vi "Configure Multi Eval Meas Modulation EVM Window Length.vi"(7 "SCS 120kHz":i32[](array[numeric]), 8 "error in (no error)":errorcluster, 9 "SCS 60kHz":i32[](array[numeric]), 10 "Instance (1)":T1=1, 11 "VISA resource name":refnum<visa-resource-name>) -> (0 "error out":errorcluster, 3 "VISA resource name out":refnum<visa-resource-name>)   [LabVIEW 2020, in "Rohde&Schwarz CMXP NR FR2 Measurement.lvlib"]
doc: "Specifies the EVM window length in samples for all channel bandwidths, depending on the SC spacing.\n\nAttribute:\nRSCMXPNRFR2M_ATTR_MULTI_EVAL_MEASUREMENT_MODULATION_EVM_WINDOW_LENGTH\n\nRemote-control command:\nCONFigure:NRMMw:MEAS<i>:MEValuation:MODulation:EWLength"
uses:
  <instrlib>/Rohde&Schwarz CMXP NR FR2 Measurement/Rohde&Schwarz CMXP NR FR2 Measurement.lvlib
  <instrlib>/Rohde&Schwarz CMXP NR FR2 Measurement/Private/_Instance.ctl
  <instrlib>/Rohde&Schwarz CMXP NR FR2 Measurement/Private/rsidr_core.llb/rsidr_core.lvlib
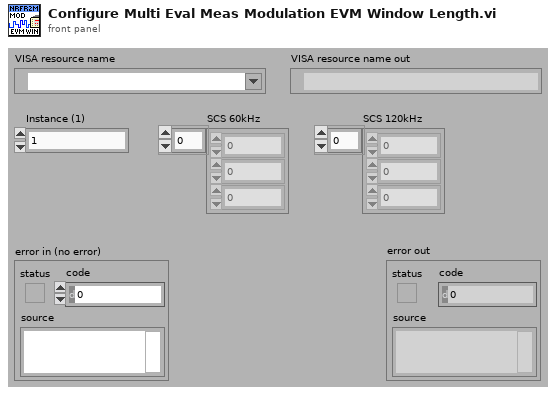
[diagram p1: front panel]
types:
  T1 = typedef "Rohde&Schwarz CMXP NR FR2 Measurement.lvlib/_Instance.ctl" = i32
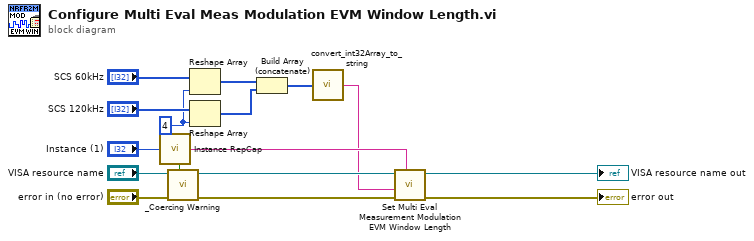
[diagram p0: block diagram]
diagram:
  w11 = 4 ("dimension size")
  n1 = call <instrlib>:"Instance RepCap.vi"("Instance In"="Instance (1)") -> ("In Range?"=w14:bool, "RepCap Identifier Out"=w6:string)  [unwired: 1 in]
  n2 = call <instrlib>:"_Coercing Warning.vi"("In Range?"=w14, "error in (no error)"="error in (no error)", "VISA resource name"="VISA resource name") -> ("error out"=w7:errorcluster, "VISA resource name out"=w8:refnum<visa-resource-name>)  [unwired: 7 in]
  n3 = Reshape Array("SCS 60kHz", w11) -> (w10:i32[])
  n4 = Reshape Array("SCS 120kHz", w11) -> (w9:i32[])
  n5 = Build Array (concatenate)(w10, w9) -> (w2:i32[])
  n6 = call <instrlib>:"convert_int32Array_to_string.vi"("I32 array in"=w2) -> ("string out"=w1:string)  [unwired: 4 in]
  n7 = call "Set Multi Eval Measurement Modulation EVM Window Length"("Repeated Capabilities"=w6, "error in (no error)"=w7, "Multi Eval Measurement Modulation EVM Window Length ()"=w1, "instrument handle"=w8) -> ("error out"=→"error out":errorcluster, "instrument handle out"=→"VISA resource name out":refnum<visa-resource-name>)  [unwired: 6 in]
